vi "SL2_AD_DLL_Phoibos_Shutdown.vi"(4 "error in":errorcluster, 6 "pHandle":u32, 7 "dll path in":path) -> (0 "error out":errorcluster, 3 "dll path out":path)   [LabVIEW 2020]
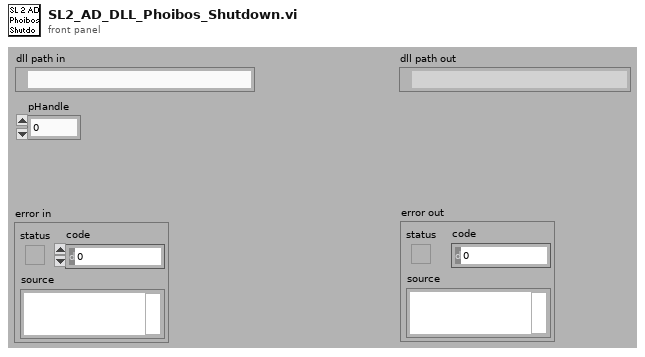
[diagram p1: front panel]
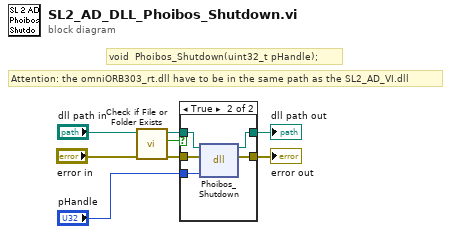
[diagram p0: block diagram]
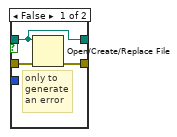
[diagram p2: hidden frame]
diagram:
  # "void  Phoibos_Shutdown(uint32_t pHandle);"
  # "Attention: the omniORB303_rt.dll have to be in the same path as the SL2_AD_VI.dll"
  n1 = call <vilib>:"Check if File or Folder Exists.vi"("error in (no error)"="error in", "path"="dll path in") -> ("error out"=w1:errorcluster, "file or folder exists?"=w3:bool, "dup path"=w2:path)  [unwired: 7 in]
  n2 = case shown="True" w3 {
    tunnel: [w10 w16] -> w8
    tunnel: [w9 w15] -> w7
    tunnel: w2 -> [w9 w14]
    tunnel: w1 -> [w11 w13]
    tunnel: "pHandle" -> [_ w12]
    frame False {
      # "only to generate an error"
      n3 = Open/Create/Replace File(file path (use dialog)=w9, error in=w11) -> (error out=w10:errorcluster)  [unwired: 4 in, 2 out]
    }
    frame True {
      n4 = dll-call lib="C:/Programme/SPECS/SpecsLab2/programming/LabView7.1/SL2_AD_VI.dll" fn="Phoibos_Shutdown"(path in=w14, error in=w13, "pHandle"=w12) -> (path out=w15:path, error out=w16:errorcluster)  [unwired: 3 in]
    }
  }
  "error out" <- w8
  "dll path out" <- w7
